vi "DMM Scan Reset.vi"(8 "error in (no error)":errorcluster, 11 "VISA in resource name":refnum<visa-resource-name>) -> (0 "error out":errorcluster, 3 "VISA resource name out":refnum<visa-resource-name>)   [LabVIEW 2023]
uses:
  <instrlib>/Agilent 3446X Series/Agilent 3446X Series.lvlib
panel:
  out "error out 4":errorcluster caption="error out"
  out "error out 3":errorcluster
  out "error out 2":errorcluster
  out "x-y":u32
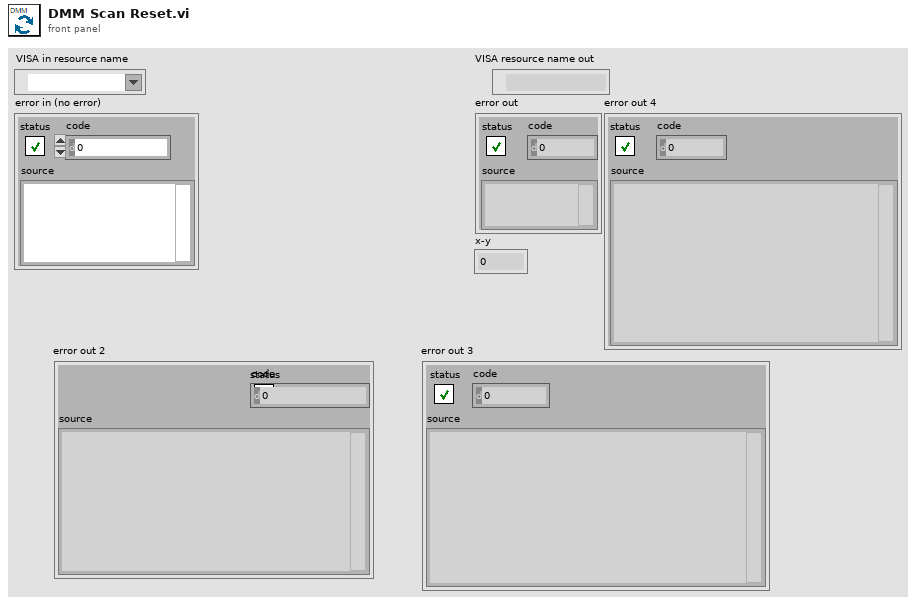
[diagram p1: front panel]
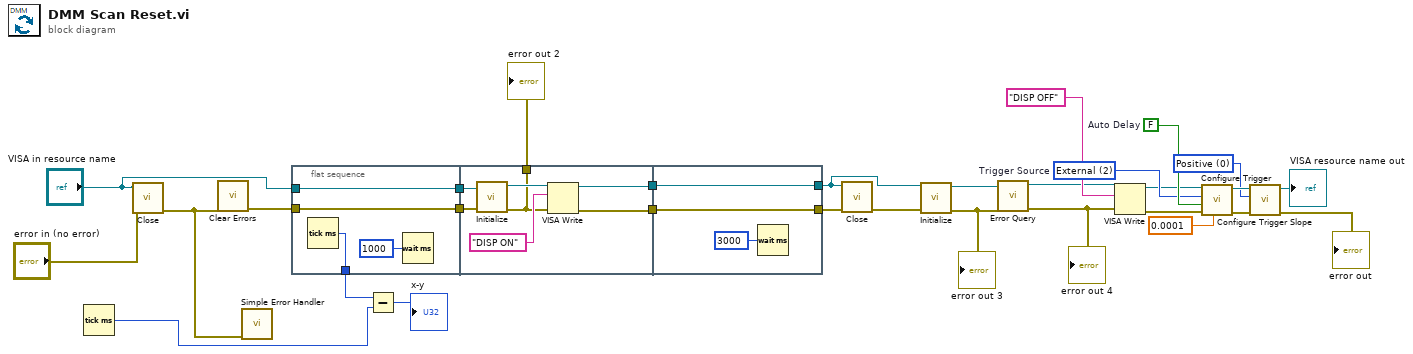
[diagram p0: block diagram]
diagram:
  w27 = 0 items=["Positive", "Negative"] ("Trigger Edge (1: Negative)")
  w25 = 2 items=["Immediate", "Software (Bus)", "External"]  # Trigger Source
  w26 = FALSE  # Auto Delay
  n1 = Tick Count (ms)() -> (millisecond timer value=w12:u32)
  n2 = call <instrlib>:"Close.vi"("error in (no error)"="error in (no error)", "VISA resource name"="VISA in resource name") -> ("error out"=w14:errorcluster)  [unwired: 9 in]
  n3 = call <vilib>:"Clear Errors.vi"("error in (no error)"=w14) -> ("error out"=w20:errorcluster)  [unwired: 5 in, 1 out]
  n4 = call <vilib>:"Simple Error Handler.vi"("error in (no error)"=w14) -> ()  [unwired: 4 in, 5 out]
  n5 = flat-sequence {
    tunnel: w20 -> [w33]
    tunnel: "VISA in resource name" -> [w34]
    tunnel: [w34] -> w16
    tunnel: [w33] -> w15
    tunnel: [w31] -> w13
    tunnel: w16 -> [w41]
    tunnel: w15 -> [w40]
    tunnel: [w36] -> w10
    tunnel: [w37] -> w9
    tunnel: [w35] -> w7
    tunnel: [w43] -> w6
    tunnel: [w44] -> w8
    tunnel: w10 -> [w44]
    tunnel: w9 -> [w43]
    frame #0 {
      n6 = Tick Count (ms)() -> (millisecond timer value=w31:u32)
      n7 = Wait (ms)(milliseconds to wait=u32 1000) -> ()  [unwired: 1 out]
    }
    frame #1 {
      n8 = call <instrlib>:"Initialize.vi"("error in (no error)"=w40, "VISA resource name"=w41) -> ("error out"=w35:errorcluster, "VISA resource name out"=w38:refnum<visa-resource-name>)  [unwired: 3 in, 5 out]
      n9 = VISA Write(VISA resource name=w38, write buffer="DISP ON", error in (no error)=w35) -> (VISA resource name out=w37:refnum<visa-resource-name>, error out=w36:errorcluster)  [unwired: 1 out]
    }
    frame #2 {
      n10 = Wait (ms)(milliseconds to wait=u32 3000) -> ()  [unwired: 1 out]
    }
  }
  n11 = Subtract(x=w13, y=w12) -> (x-y=→"x-y":u32)
  n12 = call <instrlib>:"Close.vi"("error in (no error)"=w8, "VISA resource name"=w6) -> ("error out"=w5:errorcluster)  [unwired: 9 in]
  n13 = call <instrlib>:"Initialize.vi"("error in (no error)"=w5, "VISA resource name"=w6) -> ("error out"=w3:errorcluster, "VISA resource name out"=w4:refnum<visa-resource-name>)  [unwired: 3 in, 5 out]
  "error out 3" <- w3
  n14 = call <instrlib>:"Error Query.vi"("error in (no error)"=w3, "VISA resource name"=w4) -> ("error out"=w1:errorcluster, "VISA resource name out"=w2:refnum<visa-resource-name>)  [unwired: 8 out]
  "error out 4" <- w1
  n15 = VISA Write(VISA resource name=w2, write buffer="DISP OFF", error in (no error)=w1) -> (VISA resource name out=w22:refnum<visa-resource-name>, error out=w21:errorcluster)  [unwired: 1 out]
  n16 = call <instrlib>:"Configure Trigger.vi"("Manual Trigger Delay (1 s)"=0.0001, "error in (no error)"=w21, "Auto Delay (F:Disable)"=w26, "Trigger Source (0: Immediate)"=w25, "VISA resource name"=w22) -> ("error out"=w29:errorcluster, "VISA resource name out"=w28:refnum<visa-resource-name>)  [unwired: 1 in, 4 out]
  n17 = call <instrlib>:"Configure Trigger Slope.vi"("error in (no error)"=w29, "Trigger Edge (1: Negative)"=w27, "VISA resource name"=w28) -> ("error out"=→"error out":errorcluster, "VISA resource name out"=→"VISA resource name out":refnum<visa-resource-name>)  [unwired: 7 in]
  "error out 2" <- w7
